vi "parse_header.vi"(4 "error in":errorcluster, 7 "msg in":string) -> (0 "error out":errorcluster, 2 "Header":T1, 3 "msg out":string)   [LabVIEW 2010]
uses:
  subs/parse_u32_scalar.vi
  subs/parse_time_scalar.vi
  subs/parse_string_scalar.vi
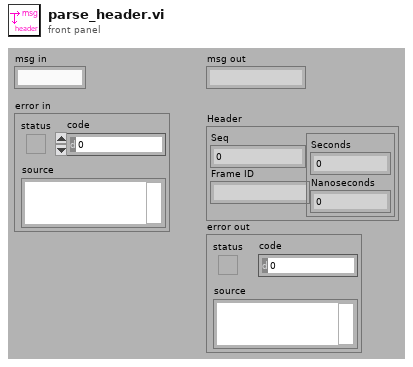
[diagram p1: front panel]
types:
  T1 = cluster{"Seq":u32, "Frame ID":string, "Timestamp":cluster{"Seconds":i32, "Nanoseconds":i32}}
  T2 = cluster{"Seq":u32, "Frame ID":string, "Time":cluster{"Seconds":i32, "Nanoseconds":i32}}
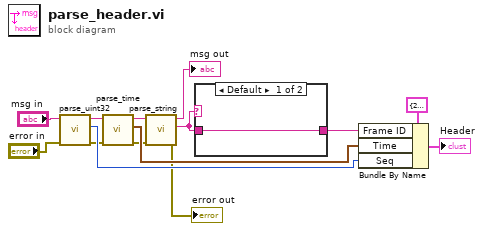
[diagram p0: block diagram]
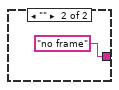
[diagram p2: hidden frame]
diagram:
  n1 = call-poly "parse_uint32.vi"("error in"="error in", "msg in"="msg in") -> ("error out"=w3:errorcluster, "number"=w9:u32, "msg out"=w14:string)  [unwired: 3 in]
  n2 = call-poly "parse_time.vi"("error in"=w3, "msg in"=w14) -> ("error out"=w4:errorcluster, "Time"=w10:cluster{"secs":i32, "nsecs":i32}, "msg out"=w13:string)  [unwired: 3 in]
  n3 = call-poly "parse_string.vi"("error in"=w4, "msg in"=w13) -> ("error out"=→"error out":errorcluster, "string"=w8:string, "msg out"=→"msg out":string)  [unwired: 3 in]
  n4 = case shown="Default" w8 {
    tunnel: [w15 "no frame" ("string")] -> w7
    tunnel: w8 -> [w15 _]
    frame Default {
    }
    frame "" {
    }
  }
  n5 = Bundle By Name(cluster=T2 {"Seq"=2284, "Frame ID"="", "Time"={"Seconds"=0, "Nanoseconds"=0}} ("ROS Msg Header"), "Frame ID"=w7, "Time"=w10, "Seq"=w9) -> (→"Header":T2)
